vi "Kinesis - KPA101 - Connect Acquire Voltage.vi"() -> ()   [LabVIEW 2013]
uses:
  C:/Users/zizhang/OneDrive - THORLABS Inc/Documents/4. SW Project/KPA101 LabVIEW/ThorLabs.MotionControl.KCube.PositionAlignerCLI.dll
  4. SW Project/KPA101 LabVIEW/ThorLabs.MotionControl.KCube.PositionAlignerCLI.dll
  C:/Users/zizhang/OneDrive - THORLABS Inc/Documents/4. SW Project/KPA101 LabVIEW/Thorlabs.MotionControl.Controls.dll
  4. SW Project/KPA101 LabVIEW/Thorlabs.MotionControl.Controls.dll
panel:
  out "SUM":dbl
  in  "Operating mode":T1(ring)
  in  "File Path":path
  in  "SerialNumber":string="69000001"
  out "Y":dbl
  out "X":dbl
  in  "stop":bool
  in  "KCubePositionAlignerControl":refnum<k24>(container)
  # "Thorlabs Hardware: KPA - K-Cube Position Sensing Detector (PSD) Auto Aligner\nhttps://www.thorlabs.com/thorproduct.cfm?partnumber=KPA101\n\nDescription: This VI will enable you to communicate with KPA101 to acquire the X, Y, and SUM voltage values. The VI will first connect to and initialize the device, set the selected operating mode, and then continuously display the X, Y, and SUM values with a default update interval of 50 ms. If a valid file path is entered, all acquired X, Y, and SUM data will be saved to the specified file when the program is stopped.\n\nInstructions: \n1) Connect your KPA101 device to your PC & power the device, ensuring your position sensing detector is connected. For full device setup, the device product manual can be found on our website here. -https://www.thorlabs.com/thorproduct.cfm?partnumber=KPA101\n2) Enter the device serial number below.\n3) Select the operating mode and, if desired, enter a valid file path for data logging.\n4) Click 'Run' in the LabVIEW toolbar. The VI will connect to the device, initialize it, and begin displaying the X, Y, and SUM values in volts.\n5) To end the program, click 'STOP'. If a valid file path was entered, all acquired X, Y, and SUM data will be automatically saved to the specified file."
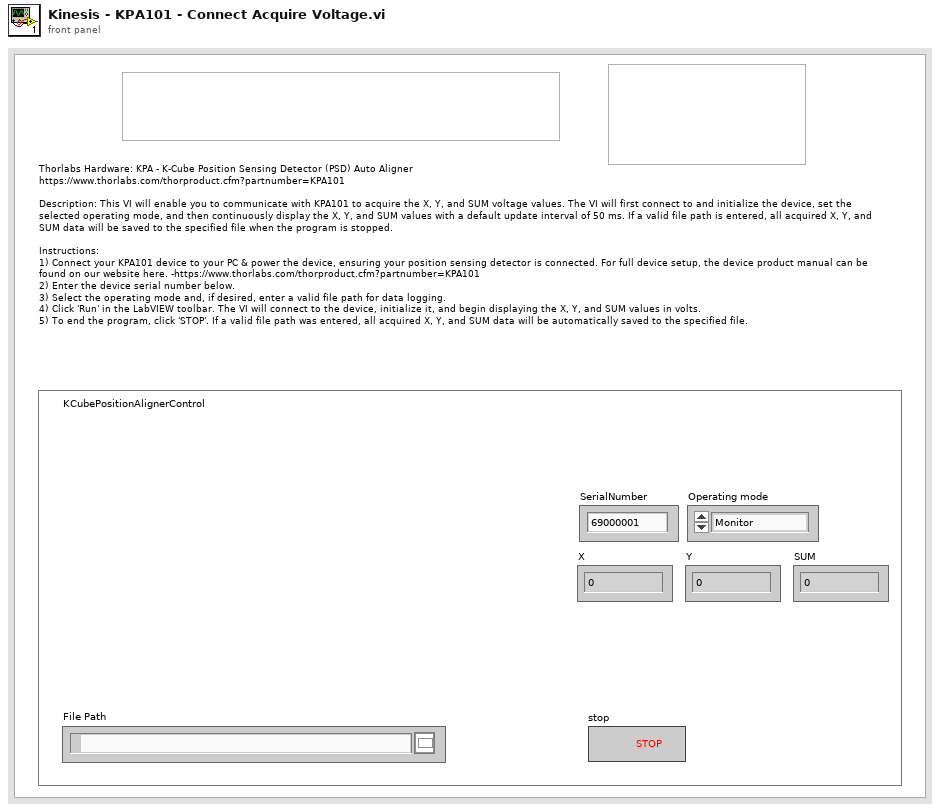
[diagram p1: front panel]
types:
  T1 = enum16{"Monitor", "OpenLoop", "ClosedLoop", "AutoOpenClosedLoop"}
  T2 = enum16{"open", "replace", "create", "open or create", "replace or create", "replace or create with confirmation"}
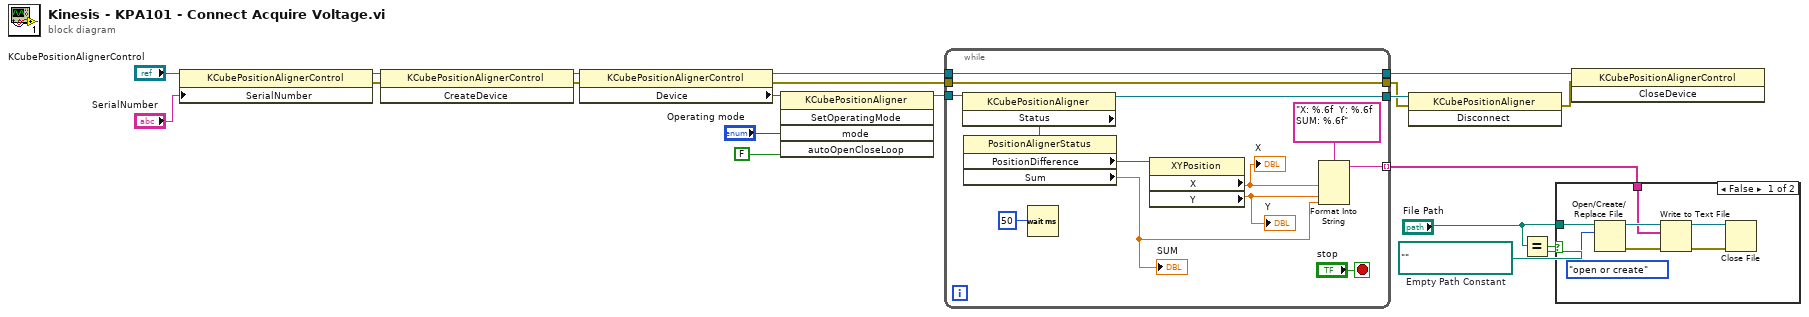
[diagram p0: block diagram]
diagram:
  w5 = path ""  # Empty Path Constant
  n1 = property class="KCubePositionAlignerControl"(reference="KCubePositionAlignerControl", "SerialNumber"="SerialNumber") -> (reference out=w19:refnum<k24>, error out=w14:errorcluster)  [unwired: 1 in]
  n2 = invoke class="KCubePositionAlignerControl" method="CreateDevice"(reference=w19, error in=w14) -> (reference out=w18:refnum<k24>, error out=w15:errorcluster)  [unwired: 1 in, 1 out]
  n3 = property class="KCubePositionAlignerControl"(reference=w18, error in=w15) -> (reference out=w16:refnum<k24>, error out=w10:errorcluster, "Device"=w13:refnum<k24>)
  n4 = invoke class="KCubePositionAligner" method="SetOperatingMode"(reference=w13, "mode"="Operating mode", "autoOpenCloseLoop"=FALSE) -> (reference out=w1:refnum<k24>)  [unwired: 2 in, 4 out]
  n5 = while {
    tunnel: w1 -> [w21]
    tunnel: [w30] -> w17
    tunnel: w16 -> [w30]
    tunnel: [w29] -> w7
    tunnel: w10 -> [w29]
    tunnel: [w28] -> w8
    tunnel: [w26] -> w4 mode=indexing
    stop <- "stop" stop-if-true
    n6 = property class="KCubePositionAligner"(reference=w21) -> (reference out=w28:refnum<k24>, "Status"=w33:refnum<k24>)  [unwired: 1 in, 1 out]
    n7 = property class="PositionAlignerStatus"(reference=w33) -> ("PositionDifference"=w25:refnum<k24>, "Sum"=w24:dbl)  [unwired: 1 in, 2 out]
    "SUM" <- w24
    n8 = Wait (ms)(milliseconds to wait=u32 50) -> ()  [unwired: 1 out]
    n9 = property class="XYPosition"(reference=w25) -> ("X"=w23:dbl, "Y"=w22:dbl)  [unwired: 1 in, 2 out]
    "X" <- w23
    "Y" <- w22
    n10 = Format Into String(format string="X: %.6f  Y: %.6f  SUM: %.6f", w23, w22, w24) -> (resulting string=w26:string)  [unwired: 2 in, 1 out]
  }
  n11 = invoke class="KCubePositionAligner" method="Disconnect"(reference=w8, error in=w7) -> (error out=w6:errorcluster)  [unwired: 1 in, 2 out]
  n12 = Equal?(x="File Path", y=w5) -> (x = y?=w3:bool)
  n13 = case shown="False" w3 {
    tunnel: w4 -> [w36 _]
    tunnel: "File Path" -> [w34 _]
    frame False {
      n14 = Open/Create/Replace File(file path (use dialog)=w34, operation (0:open)=T2."open or create") -> (refnum out=w39:refnum<file>, error out=w40:errorcluster)  [unwired: 4 in, 1 out]
      n15 = Write to Text File(file (use dialog)=w39, text=w36, error in=w40) -> (refnum out=w37:refnum<file>, error out=w38:errorcluster)  [unwired: 1 in, 1 out]
      n16 = Close File(refnum=w37, error in=w38) -> ()  [unwired: 2 out]
    }
    frame True {
    }
  }
  n17 = invoke class="KCubePositionAlignerControl" method="CloseDevice"(reference=w17, error in=w6) -> ()  [unwired: 1 in, 3 out]
